vi "ClimberBegin.vi"(8 "error in (no error)":errorcluster, 10 "Configuration In":variant, 11 "ScissorClimber in":refnum<class "ScissorClimber.lvclass">) -> (0 "error out":errorcluster, 3 "ScissorClimber out":refnum<class "ScissorClimber.lvclass">)   [LabVIEW 2019, in "Climber.lvlib" / "ScissorClimber.lvclass"]
uses:
  ScissorClimber.lvclass
  <vilib>/Rock Robotics/WPI/ThirdParty/Phoenix-LabVIEW/Motor Controller/Controls/CTRE_Phoenix_MotorControl_FeedbackDevice_TalonFX.ctl
  Climber.lvclass
  <vilib>/Rock Robotics/WPI/ThirdParty/Phoenix-LabVIEW/Motor Controller/Controls/CTRE_Phoenix_MotorControl_TalonFXInvertType.ctl
  Drive/Tank Drive/Controls/PIDF.ctl
  Drive/Tank Drive/Tank Drive.lvclass
  <vilib>/Rock Robotics/WPI/ThirdParty/Phoenix-LabVIEW/Motor Controller/Controls/CTRE_Phoenix_MotorControl_SupplyCurrentLimitConfiguration.ctl
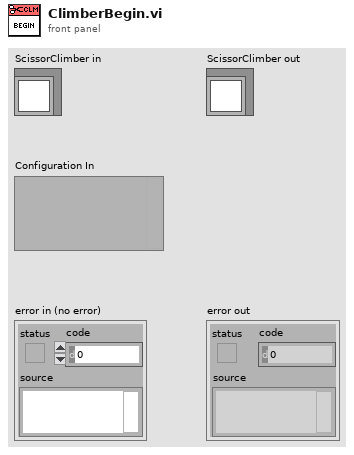
[diagram p1: front panel]
types:
  T1 = typedef "CTRE_Phoenix_MotorControl_SupplyCurrentLimitConfiguration.ctl" = cluster{"Enable?":bool, "Current Limit":dbl, "Threshold Current":dbl, "Threshold Time":dbl}
  T2 = typedef "Drive.lvlib/Tank Drive.lvclass/PIDF.ctl" = cluster{"P":dbl, "I":dbl, "D":dbl, "F":dbl}
  T3 = typedef "CTRE_Phoenix_MotorControl_FeedbackDevice_TalonFX.ctl" = i8
  T4 = typedef "Climber.lvlib/Climber.lvclass/Screw Motor.ctl" = cluster{"Refnum Name":string, "CAN ID":u32, "I":dbl, "D":dbl, "P":dbl, "F":dbl, "Velocity":dbl, "Acceleration":dbl}
  T5 = typedef "WPI_MotorControlDeviceRef.ctl" = cluster{"DeviceStatus":errorcluster, "Type":T6, "PWM":cluster{"PWM Channel":T7, "DeadBand":T8}, "CAN":cluster{"Device Number":u8, "SetOutput VI Ref":variant, "GetOutput VI Ref":variant, "Enable VI Ref":variant, "Disable VI Ref":variant, "Data":variant}, "Invert":bool, "DIO PWM":cluster{"PWM \"Enable\" Channel":T7, "DIOChannel":T9, "PWM Rate":dbl}}
  T6 = typedef "WPI_MotorControlType.ctl" = enum16{"PWM", "CAN", "DIO PWM"}
  T7 = typedef "FPGA_DIOPWMChannel.ctl" = enum8{"PWM 0", "PWM 1", "PWM 2", "PWM 3", "PWM 4", "PWM 5", "PWM 6", "PWM 7", "PWM 8", "PWM 9", "PWM MXP 0", "PWM MXP 1", "PWM MXP 2", "PWM MXP 3", "PWM MXP 4", "PWM MXP 5", "PWM MXP 6", "PWM MXP 7", "PWM MXP 8", "PWM MXP 9", "Invalid"}
  T8 = typedef "WPI_PWMDeadband.ctl" = cluster{"Name":string, "maxPositivePwm":i32, "minPositivePwm":i32, "centerPwm":i32, "maxNegativePwm":i32, "minNegativePwm":i32, "angularRange":u16}
  T9 = typedef "FPGA_DIOChannel.ctl" = enum8{"DIO 0", "DIO 1", "DIO 2", "DIO 3", "DIO 4", "DIO 5", "DIO 6", "DIO 7", "DIO 8", "DIO 9", "DIO MXP 0", "DIO MXP 1", "DIO MXP 2", "DIO MXP 3", "DIO MXP 4", "DIO MXP 5", "DIO MXP 6", "DIO MXP 7", "DIO MXP 8", "DIO MXP 9", "DIO MXP 10", "DIO MXP 11", "DIO MXP 12", "DIO MXP 13", "DIO MXP 14", "DIO MXP 15", "SPI Port CS1", "SPI Port CS2", "SPI Port CS3", "SPI Port MISO", "SPI Port MOSI", "Invalid"}
  T10 = typedef "CTRE_Phoenix_MotorControl_TalonFXInvertType.ctl" = enum16{"Counter-Clockwise", "Clockwise"}
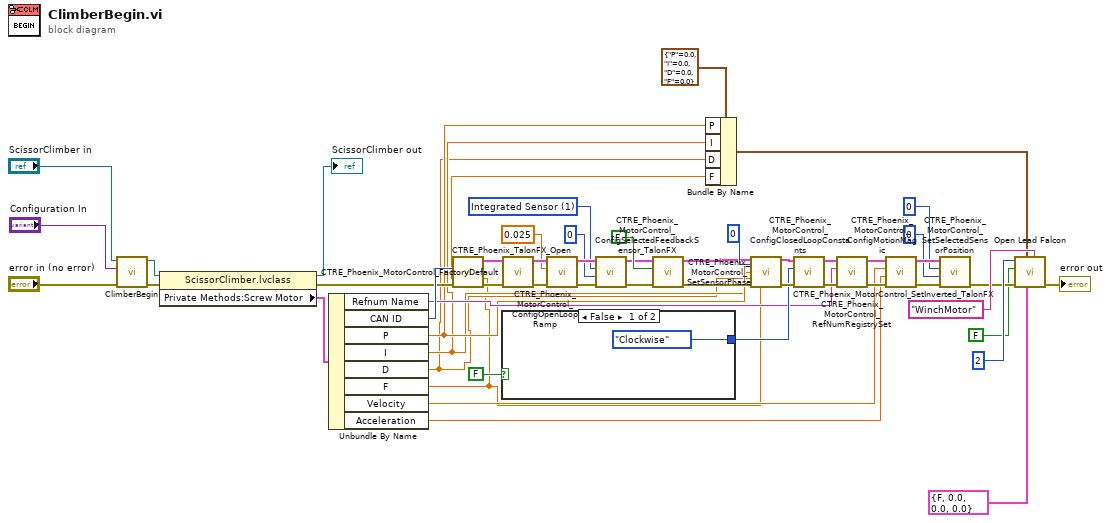
[diagram p0: block diagram]
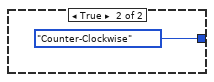
[diagram p2: hidden frame]
diagram:
  w10 = T3 1 items=["Integrated Sensor"=1, "Sensor Sum (S0 + S1)"=9, "Sensor Difference (D0 - D1)"=10, "Remote Source 0"=11, "Remote Source 1"=12, "None"=14, "Software Emulated"=15] ("Talon FX Feedback Device")
  n1 = call-parent "ClimberBegin.vi"("error in (no error)"="error in (no error)", "Configuration In"="Configuration In", "Climber in"="ScissorClimber in") -> ("error out"=w37:errorcluster, "Climber out"=w32:refnum<class "ScissorClimber.lvclass">)  [unwired: 7 in]
  n2 = property class="ScissorClimber.lvclass"(reference=w32, error in=w37) -> (reference out=→"ScissorClimber out":refnum<class "ScissorClimber.lvclass">, error out=w33:errorcluster, "Private Methods:Screw Motor"=w31:T4)
  n3 = Unbundle By Name(w31) -> ("Refnum Name"=w9:string, "CAN ID"=w41:u32, "P"=w6:dbl, "I"=w5:dbl, "D"=w4:dbl, "F"=w3:dbl, "Velocity"=w40:dbl, "Acceleration"=w39:dbl)
  n4 = call <vilib>:"CTRE_Phoenix_TalonFX_Open.vi"("error in"=w33, "Device Number"=w41) -> ("error out"=w11:errorcluster, "CAN Talon SRX Ref"=w12:T5)  [unwired: 8 in]
  n5 = case shown="False" FALSE ("Invert") {
    tunnel: [CTRE_Phoenix_MotorControl_TalonFXInvertType."Clockwise" ("Invert Type") CTRE_Phoenix_MotorControl_TalonFXInvertType."Counter-Clockwise" ("Invert Type")] -> w23
    frame False {
    }
    frame True {
    }
  }
  n6 = call <vilib>:"CTRE_Phoenix_MotorControl_FactoryDefault.vi"("error in"=w11, "PhoenixMotorControlDevRef"=w12) -> ("error out"=w18:errorcluster, "PhoenixMotorControlDevRef"=w17:T5)  [unwired: 8 in]
  n7 = call <vilib>:"CTRE_Phoenix_MotorControl_ConfigOpenLoopRamp.vi"("error in (no error)"=w18, "secondsFromNeutralToFull"=0.025, "PhoenixMotorControlDevRef"=w17) -> ("error out"=w20:errorcluster, "PhoenixMotorControlDevRef"=w19:T5)  [unwired: 7 in]
  n8 = call <vilib>:"CTRE_Phoenix_MotorControl_ConfigSelectedFeedbackSensor_TalonFX.vi"("error in (no error)"=w20, "pidLoopIdx"=0, "Talon FX Feedback Device"=w10, "PhoenixMotorControlDevRef"=w19) -> ("error out"=w15:errorcluster, "PhoenixMotorControlDevRef"=w14:T5)  [unwired: 6 in]
  n9 = call <vilib>:"CTRE_Phoenix_MotorControl_SetSensorPhase.vi"("error in (no error)"=w15, "PhaseSensor"=FALSE, "PhoenixMotorControlDevRef"=w14) -> ("error out"=w25:errorcluster, "PhoenixMotorControlDevRef"=w24:T5)  [unwired: 7 in]
  n10 = Bundle By Name(cluster=T2 {"P"=0.0, "I"=0.0, "D"=0.0, "F"=0.0} ("PIDF Constants"), "P"=w6, "I"=w5, "D"=w4, "F"=w3) -> (w2:T2)
  n11 = call <vilib>:"CTRE_Phoenix_MotorControl_ConfigClosedLoopConstants.vi"("PhoenixMotorControlDevRef"=w24, "slotIdx"=0, "P"=w6, "I"=w5, "D"=w4, "error in (no error)"=w25, "F"=w3) -> ("PhoenixMotorControlDevRef"=w26:T5, "error out"=w27:errorcluster)  [unwired: 7 in]
  n12 = call <vilib>:"CTRE_Phoenix_MotorControl_SetInverted_TalonFX.vi"("error in (no error)"=w27, "Invert Type"=w23, "PhoenixMotorControlDevRef"=w26) -> ("error out"=w21:errorcluster, "PhoenixMotorControlDevRef"=w22:T5)  [unwired: 7 in]
  n13 = call <vilib>:"CTRE_Phoenix_MotorControl_RefNumRegistrySet.vi"("error in (no error)"=w21, "refnum name"=w9, "PhoenixMotorControlDevRef"=w22) -> ("error out"=w46:errorcluster, "PhoenixMotorControlDevRef"=w47:T5)  [unwired: 7 in]
  n14 = call <vilib>:"CTRE_Phoenix_MotorControl_ConfigMotionMagic.vi"("error in (no error)"=w46, "Acceleration"=w39, "Cruise Velocity"=w40, "PhoenixMotorControlDevRef"=w47) -> ("error out"=w36:errorcluster, "PhoenixMotorControlDevRef"=w44:T5)  [unwired: 6 in]
  n15 = call <vilib>:"CTRE_Phoenix_MotorControl_SetSelectedSensorPosition.vi"("error in (no error)"=w36, "pidLoopIdx"=u32 0, "New Sensor Position"=0, "PhoenixMotorControlDevRef"=w44) -> ("error out"=w35:errorcluster)  [unwired: 6 in, 1 out]
  n16 = call "Open Lead Falcon.vi"("refnum name"="WinchMotor", "Supply Current Limit Configuration"=T1 {"Enable?"=FALSE, "Current Limit"=0.0, "Threshold Current"=0.0, "Threshold Time"=0.0}, "PIDF Constants"=w2, "error in (no error)"=w35, "Drive Invert"=FALSE ("Invert"), "can id"=u8 2) -> ("error out"=→"error out":errorcluster)  [unwired: 4 in, 1 out]
